vi "Facade 1.vi"(0 "Data In":T5, 2 "Display State In":T3, 3 "Container State":T4) -> (6 "Data Out":T5, 7 "Display State Out":T3, 8 "Action":T2)   [LabVIEW 2017, in "Selection.xctl"]
uses:
  Selection.xctl
  Data 1.ctl
  Signal types.ctl
  <vilib>/_xctls/Container State.ctl
  State 1.ctl
  <vilib>/_xctls/Action.ctl
  <vilib>/_xctls/XControlSupport.lvlib
panel:
  in  "Index 2":i32 min=0
  in  "Index 1":i32 min=0
  in  "Type":T1
  in  "Index":i32 min=0
  # "1. Drop the controls that make up the appearance\nof the XControl here.\n\n2. Resize the window to fit the controls\n\n3. If the XControl is of fixed size,  make the \n window not resizable from VI Properties->Window Appearance.\n\n4. If you want the controls to automatically size when the XControl sizes, check  \"Scale all objects on front panel when window resizes\" in File->VI Properties->Window Size page.\n\n5. Show the block diagram and handle events for the controls on this panel."
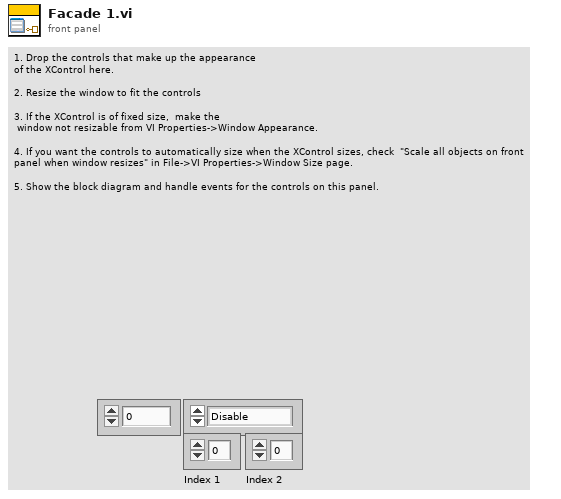
[diagram p1: front panel]
types:
  T1 = typedef "Selection.xctl/Signal types.ctl" = enum16{"Disable", "Frequency", "Phasor Mag", "Phasor Ang", "Angle Diff", "P", "Q"}
  T2 = typedef "XControlSupport.lvlib/Action.ctl" = cluster{"Data Changed?":bool, "State Changed?":bool, "Action Name":string}
  T3 = typedef "Selection.xctl/State 1.ctl" = cluster{"Numeric":dbl}
  T4 = typedef "XControlSupport.lvlib/Container State.ctl" = cluster{"Indicator?":bool, "Run Mode?":bool, " Refnum":refnum<vi>}
  T5 = typedef "Selection.xctl/Data 1.ctl" = cluster{"Type":T1, "Index(es)":i32[]}[]
  T6 = enum8{"Enabled", "Disabled", "Disabled and Grayed Out"}
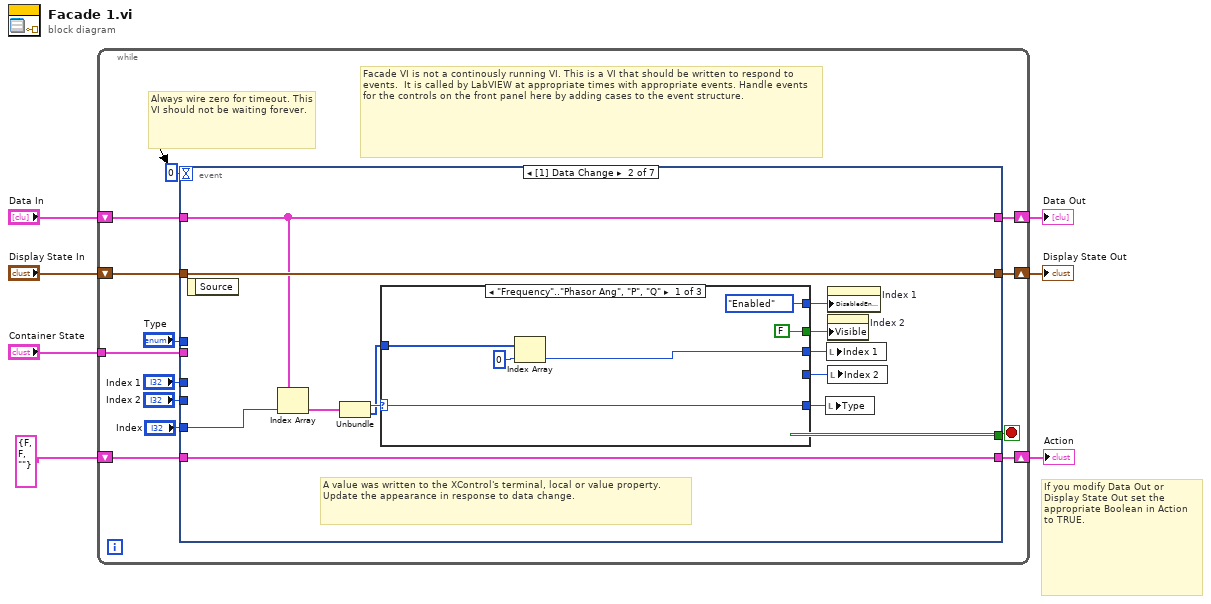
[diagram p0: block diagram]
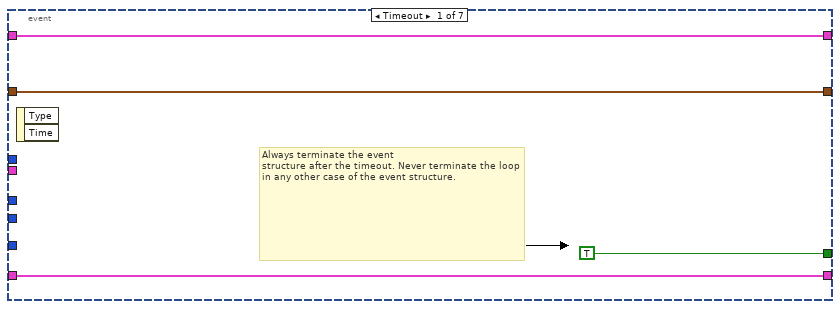
[diagram p2: hidden frame]
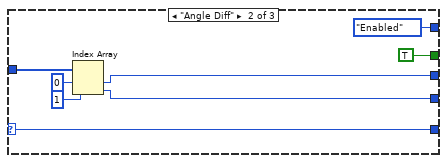
[diagram p3: hidden frame]
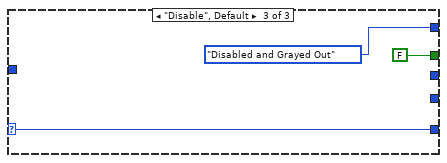
[diagram p4: hidden frame]
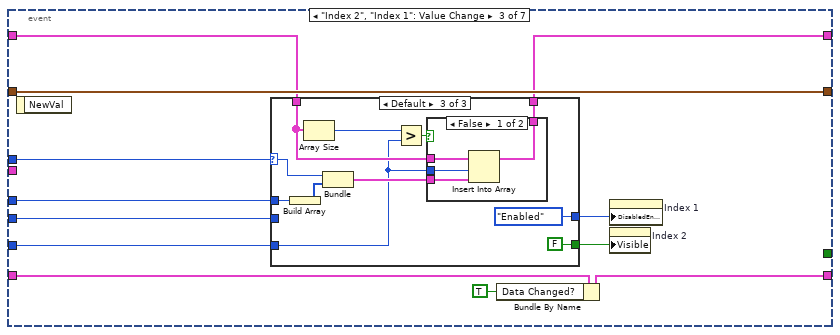
[diagram p5: hidden frame]
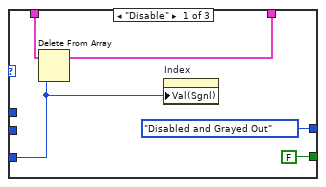
[diagram p6: hidden frame]
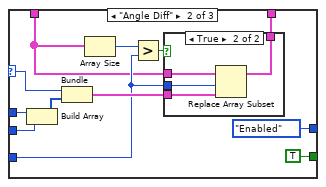
[diagram p7: hidden frame]
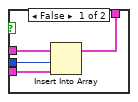
[diagram p8: hidden frame]
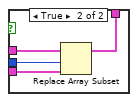
[diagram p9: hidden frame]
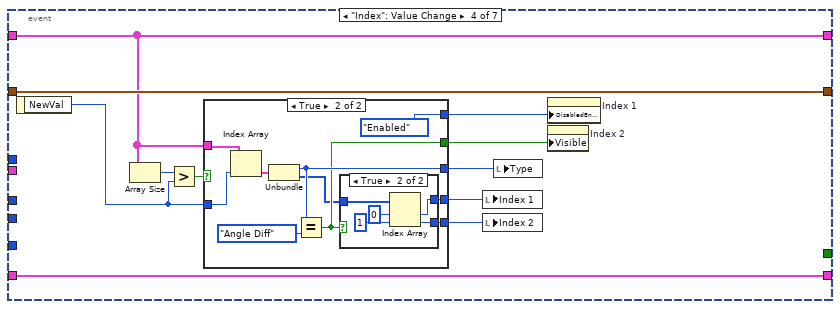
[diagram p10: hidden frame]
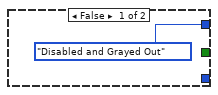
[diagram p11: hidden frame]
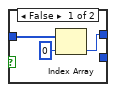
[diagram p12: hidden frame]
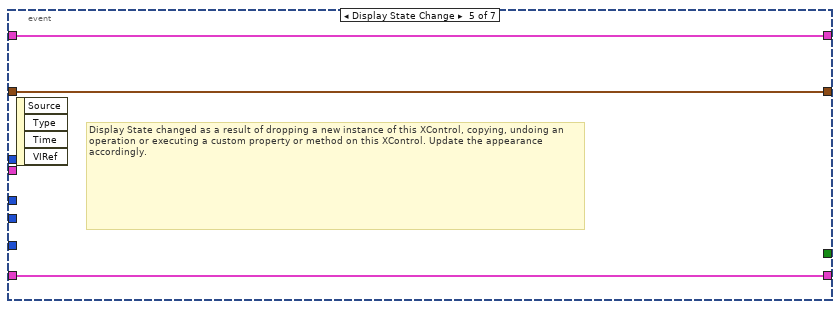
[diagram p13: hidden frame]
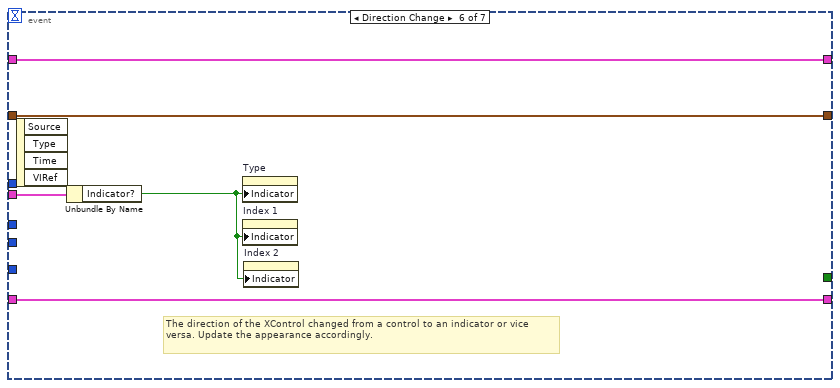
[diagram p14: hidden frame]
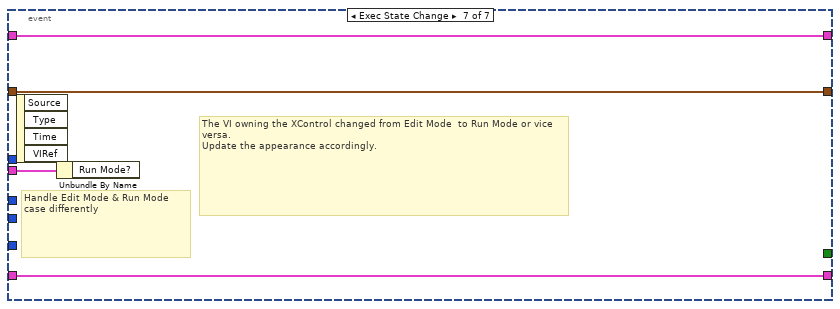
[diagram p15: hidden frame]
diagram:
  # "If you modify Data Out or\nDisplay State Out set the\nappropriate Boolean in Action\nto TRUE."
  n1 = while {
    shift-right: [w19] -> w4
    shift-left: "Display State In" -> [w20]
    tunnel: "Container State" -> [w16]
    shift-right: [w8] -> w7
    shift-left: "Data In" -> [w9]
    shift-right: [w14] -> w2
    shift-left: T2 {"Data Changed?"=FALSE, "State Changed?"=FALSE, "Action Name"=""} ("Action") -> [w15]
    stop <- w18 stop-if-true
    # "Facade VI is not a continously running VI. This is a VI that should be written to respond to events.  It is called by LabVIEW at appropriate times with appropriate events. Handle events for the controls on the front panel here by adding cases to the event structure."
    # "Always wire zero for timeout. This\nVI should not be waiting forever."
    n2 = event shown="[1] Data Change" {
      selector: _ -> [_ _ _ _ _ _ _]
      dyn-events: _ -> [_ _ _ _ _ _ _]
      timeout: 0 -> [_ _ _ _ _ _ _]
      tunnel: w20 -> [w22 w36 w65 w120 w142 w146 w150]
      tunnel: [w22 w36 w65 w120 w142 w146 w150] -> w19
      tunnel: [TRUE _ _ _ _ _ _] -> w18
      tunnel: w16 -> [_ _ _ _ _ w147 w151]
      tunnel: w9 -> [w21 w33 w59 w118 w141 w145 w149]
      tunnel: [w21 w33 w56 w118 w141 w145 w149] -> w8
      tunnel: [w23 w35 w61 w119 w140 w144 w148] -> w14
      tunnel: w15 -> [w23 w35 w62 w119 w140 w144 w148]
      tunnel: "Index" -> [_ w32 w57 _ _ _ _]
      tunnel: "Type" -> [_ _ w58 _ _ _ _]
      tunnel: "Index 2" -> [_ _ w63 _ _ _ _]
      tunnel: "Index 1" -> [_ _ w64 _ _ _ _]
      event Timeout {
        # "Always terminate the event\nstructure after the timeout. Never terminate the loop in any other case of the event structure."
        n3 = event-data() -> ()  [unwired: 1 in, 2 out]
      }
      event Data Change {
        # "A value was written to the XControl's terminal, local or value property.\nUpdate the appearance in response to data change."
        n4 = event-data() -> ()  [unwired: 1 in, 1 out]
        n5 = Index Array(array=w33, index=w32) -> (element=w34:cluster{"Type":T1, "Index(es)":i32[]})
        n6 = Unbundle(w34) -> ("Type"=w31:T1, "Index(es)"=w30:i32[])
        n7 = case shown="\"Frequency\"..\"Phasor Ang\", \"P\", \"Q\"" w31 {
          selector: w31 -> [w39 w49 w52]
          tunnel: [FALSE ("Visible") TRUE ("Visible") FALSE ("Visible")] -> w26
          tunnel: w30 -> [w41 w48 _]
          tunnel: [w39 w49 w52] -> w29
          tunnel: [w38 w45 _] -> w28
          tunnel: [_ w44 _] -> w27
          tunnel: [T6."Enabled" ("Disabled") T6."Enabled" ("Disabled") T6."Disabled and Grayed Out" ("Disabled")] -> w25
          frame "Frequency".."Phasor Ang", "P", "Q" {
            n8 = Index Array(array=w41, index=0) -> (element=w38:i32)
          }
          frame "Angle Diff" {
            n9 = Index Array(array=w48, index #1=0 ("index"), index #2=1 ("index")) -> (element #1=w45:i32, element #2=w44:i32)
          }
          frame "Disable", Default {
          }
        }
        n10 = local write "Type"(w29) -> ()
        n11 = local write "Index 1"(w28) -> ()
        n12 = property on="Index 1" class="DigNum (strict)"("DisabledEnum"=w25) -> ()  [unwired: 2 in, 2 out]
        n13 = property on="Index 2" class="DigNum (strict)"("Visible"=w26) -> ()  [unwired: 2 in, 2 out]
        n14 = local write "Index 2"(w27) -> ()
      }
      event "Index 2", "Index 1": Value Change {
        n15 = event-data() -> ()  [unwired: 1 in, 1 out]
        n16 = case shown="Default" w58 {
          selector: w58 -> [_ w82 w98]
          tunnel: w64 -> [_ w81 w99]
          tunnel: w63 -> [_ w80 _]
          tunnel: [w69 w73 w100] -> w56
          tunnel: w59 -> [w70 w74 w96]
          tunnel: w57 -> [w66 w76 w93]
          tunnel: [T6."Disabled and Grayed Out" ("Disabled") T6."Enabled" ("Disabled") T6."Enabled" ("Disabled")] -> w55
          tunnel: [FALSE ("Data Changed?") TRUE ("Data Changed?") FALSE ("Data Changed?")] -> w54
          frame "Disable" {
            n17 = Delete From Array(array=w70, index=w66) -> (array with subset deleted=w69:T5)  [unwired: 1 in, 1 out]
            n18 = property on="Index" class="DigNum (strict)"("Val(Sgnl)"=w66) -> ()  [unwired: 2 in, 2 out]
          }
          frame "Angle Diff" {
            n19 = Build Array(w81, w80) -> (w79:i32[])
            n20 = Bundle("Type"=w82, w79) -> (w77:cluster{"Type":T1, i32[]})  [unwired: 1 in]
            n21 = Array Size(array=w74) -> (size(s)=w75:i32)
            n22 = Greater?(x=w75, y=w76) -> (0:w78:bool)
            n23 = case shown="True" w78 {
              tunnel: w74 -> [w86 w90]
              tunnel: [w85 w89] -> w73
              tunnel: w77 -> [w84 w88]
              tunnel: w76 -> [w83 w87]
              frame False {
                n24 = Insert Into Array(array=w86, index=w83, new element=w84) -> (w85:T5)
              }
              frame True {
                n25 = Replace Array Subset(array=w90, new element=w88, index=w87) -> (w89:T5)
              }
            }
          }
          frame Default {
            n26 = Build Array(w99) -> (w101:i32[])
            n27 = Array Size(array=w96) -> (size(s)=w95:i32)
            n28 = Bundle("Type"=w98, w101) -> (w97:cluster{"Type":T1, i32[]})  [unwired: 1 in]
            n29 = Greater?(x=w95, y=w93) -> (0:w94:bool)
            n30 = case shown="False" w94 {
              tunnel: w96 -> [w105 w109]
              tunnel: [w104 w108] -> w100
              tunnel: w97 -> [w103 w107]
              tunnel: w93 -> [w102 w106]
              frame False {
                n31 = Insert Into Array(array=w105, index=w102, new element=w103) -> (w104:T5)
              }
              frame True {
                n32 = Replace Array Subset(array=w109, new element=w107, index=w106) -> (w108:T5)
              }
            }
          }
        }
        n33 = Bundle By Name(cluster=w62, "Data Changed?"=TRUE) -> (w61:T2)
        n34 = property on="Index 1" class="DigNum (strict)"("DisabledEnum"=w55) -> ()  [unwired: 2 in, 2 out]
        n35 = property on="Index 2" class="DigNum (strict)"("Visible"=w54) -> ()  [unwired: 2 in, 2 out]
      }
      event "Index": Value Change {
        n36 = event-data() -> ("NewVal"=w110:i32)  [unwired: 1 in]
        n37 = Array Size(array=w118) -> (size(s)=w117:i32)
        n38 = Greater?(x=w117, y=w110) -> (0:w116:bool)
        n39 = case shown="True" w116 {
          tunnel: w110 -> [_ w131]
          tunnel: w118 -> [_ w130]
          tunnel: [_ w127] -> w115
          tunnel: [_ w125] -> w114
          tunnel: [T6."Disabled and Grayed Out" ("Disabled") T6."Enabled" ("Disabled")] -> w113
          tunnel: [_ w123] -> w112
          tunnel: [_ w122] -> w111
          frame False {
          }
          frame True {
            n40 = Index Array(array=w130, index=w131) -> (element=w129:cluster{"Type":T1, "Index(es)":i32[]})
            n41 = Unbundle(w129) -> ("Type"=w127:T1, "Index(es)"=w124:i32[])
            n42 = Equal?(x=w127, y=Signal_types."Angle Diff" ("Type")) -> (x = y?=w125:bool)
            n43 = case shown="True" w125 {
              tunnel: w124 -> [w133 w139]
              tunnel: [w132 w136] -> w123
              tunnel: [_ w135] -> w122
              frame False {
                n44 = Index Array(array=w133, index=0) -> (element=w132:i32)
              }
              frame True {
                n45 = Index Array(array=w139, index #1=0 ("index"), index #2=1 ("index")) -> (element #1=w136:i32, element #2=w135:i32)
              }
            }
          }
        }
        n46 = local write "Index 1"(w112) -> ()
        n47 = local write "Index 2"(w111) -> ()
        n48 = local write "Type"(w115) -> ()
        n49 = property on="Index 1" class="DigNum (strict)"("DisabledEnum"=w113) -> ()  [unwired: 2 in, 2 out]
        n50 = property on="Index 2" class="DigNum (strict)"("Visible"=w114) -> ()  [unwired: 2 in, 2 out]
      }
      event Display State Change {
        # "Display State changed as a result of dropping a new instance of this XControl, copying, undoing an operation or executing a custom property or method on this XControl. Update the appearance accordingly."
        n51 = event-data() -> ()  [unwired: 1 in, 4 out]
      }
      event Direction Change {
        # "The direction of the XControl changed from a control to an indicator or vice versa. Update the appearance accordingly."
        n52 = event-data() -> ()  [unwired: 1 in, 4 out]
        n53 = Unbundle By Name(w147) -> ("Indicator?"=w143:bool)
        n54 = property on="Type" class="Enum (strict)"("Indicator"=w143) -> ()  [unwired: 2 in, 2 out]
        n55 = property on="Index 1" class="DigNum (strict)"("Indicator"=w143) -> ()  [unwired: 2 in, 2 out]
        n56 = property on="Index 2" class="DigNum (strict)"("Indicator"=w143) -> ()  [unwired: 2 in, 2 out]
      }
      event Exec State Change {
        # "The VI owning the XControl changed from Edit Mode  to Run Mode or vice versa.\nUpdate the appearance accordingly."
        # "Handle Edit Mode & Run Mode\ncase differently"
        n57 = event-data() -> ()  [unwired: 1 in, 4 out]
        n58 = Unbundle By Name(w151) -> ()  [unwired: 1 out]
      }
    }
  }
  "Display State Out" <- w4
  "Data Out" <- w7
  "Action" <- w2
